vi "TBQ_EnforceMaximumAge.vi"(11 "TimeBasedQueue In":refnum<class "TimeBasedQueue.lvclass">) -> (3 "TimeBasedQueue Out":refnum<class "TimeBasedQueue.lvclass">)   [LabVIEW 2012, in "TimeBasedQueue.lvclass"]
uses:
  TimeBasedQueue.lvclass
  TimeBasedQueue.lvclass/TimeBasedQueue.ctl
panel:
  out "Array":dbl[](array[numeric])
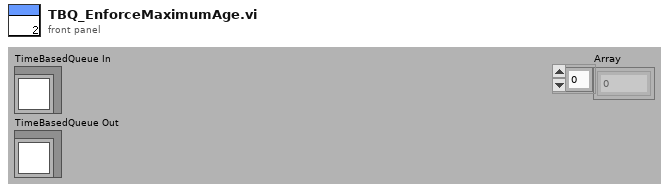
[diagram p1: front panel]
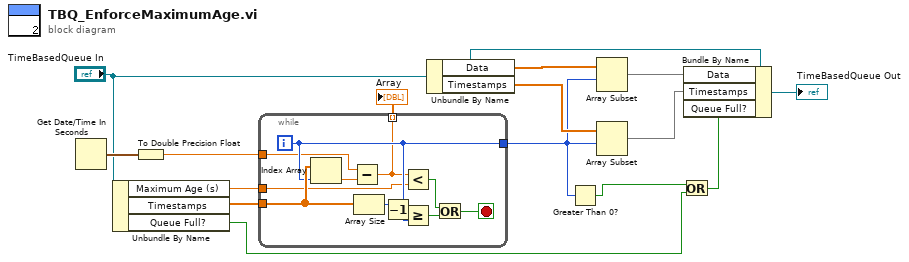
[diagram p0: block diagram]
diagram:
  n1 = Get Date/Time In Seconds() -> (seconds since 1Jan1904=w14:timestamp)
  n2 = Unbundle By Name("TimeBasedQueue In") -> ("Maximum Age (s)"=w12:dbl, "Timestamps"=w15:dbl[], "Queue Full?"=w4:bool)
  n3 = To Double Precision Float(number=w14) -> (double precision float=w13:dbl)
  n4 = while {
    tunnel: w15 -> [w24]
    tunnel: w13 -> [w21]
    tunnel: w12 -> [w19]
    tunnel: [w23] -> w2
    tunnel: [w17] -> w3 mode=indexing
    i -> [w23]
    stop <- w25 stop-if-true
    n5 = Index Array(array=w24, index=w23) -> (element=w20:dbl)
    n6 = Subtract(x=w21, y=w20) -> (x-y=w17:dbl)
    n7 = Array Size(array=w24) -> (size(s)=w22:i32)
    n8 = Decrement(x=w22) -> (x-1=w16:i32)
    n9 = Less?(x=w17, y=w19) -> (x < y?=w18:bool)
    n10 = Greater Or Equal?(x=w23, y=w16) -> (x >= y?=w26:bool)
    n11 = Or(x=w18, y=w26) -> (x .or. y?=w25:bool)
  }
  "Array" <- w3
  n12 = Unbundle By Name("TimeBasedQueue In") -> ("Data"=w11:dbl[], "Timestamps"=w6:dbl[])
  n13 = Greater Than 0?(x=w2) -> (x > 0?=w1:bool)
  n14 = Array Subset(array=w11, index=w2) -> (w9:dbl[])  [unwired: 1 in]
  n15 = Array Subset(array=w6, index=w2) -> (w8:dbl[])  [unwired: 1 in]
  n16 = Or(x=w1, y=w4) -> (x .or. y?=w5:bool)
  n17 = Bundle By Name(cluster="TimeBasedQueue In", "Data"=w9, "Timestamps"=w8, "Queue Full?"=w5) -> (→"TimeBasedQueue Out":refnum<class "TimeBasedQueue.lvclass">)
